vi "Memory.Pointer.Dispose.vi"(8 "error in (no error)":errorcluster, 11 "Pointer in":refnum<class "Memory.Pointer.lvclass">) -> (0 "error out":errorcluster)   [LabVIEW 2016, in "LabVIEW Memory Manager.lvlib" / "Memory.Pointer.lvclass"]
uses:
  Memory.Pointer.lvclass
  Memory.Pointer.lvclass/Memory.Pointer.ctl
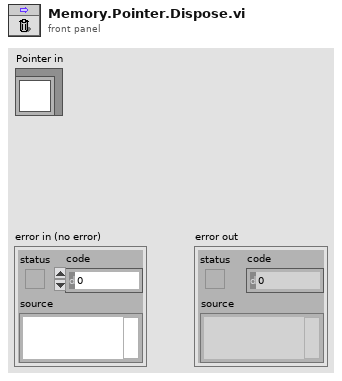
[diagram p1: front panel]
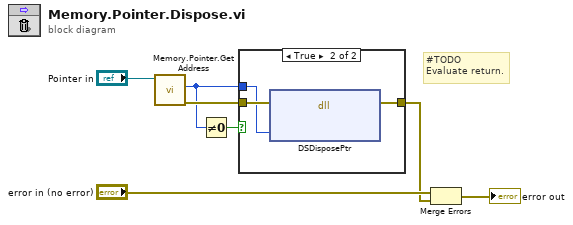
[diagram p0: block diagram]
diagram:
  # "#TODO\nEvaluate return."
  n1 = call "Memory.Pointer.Get Address.vi"("Pointer in"="Pointer in") -> ("error out"=w6:errorcluster, "address"=w5:u64)  [unwired: 8 in, 1 out]
  n2 = Not Equal To 0?(x=w5) -> (x != 0?=w4:bool)
  n3 = case shown="True" w4 {
    tunnel: w6 -> [w8 w11]
    tunnel: [w8 w10] -> w2
    tunnel: w5 -> [_ w9]
    frame False {
    }
    frame True {
      n4 = dll-call lib="LabVIEW" fn="DSDisposePtr"(error in=w11, "pointer"=w9) -> (error out=w10:errorcluster)  [unwired: 4 in, 1 out]
    }
  }
  n5 = Merge Errors("error in (no error)", w2) -> (→"error out":errorcluster)
